vi "ptr_write.vi"() -> ()   [LabVIEW 2013]
panel:
  in  "ptr_write":i32
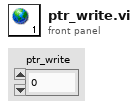
[diagram p1: front panel]
diagram:
